vi "Select Script Mode and Run Script.vi"(7 "script name":string, 8 "error in (no error)":errorcluster, 11 "Semiconductor Module Context":T1) -> (0 "error out":errorcluster, 2 "HSDIO GEN Sessions Out":refnum<k15>[](array[refnum]), 3 "Semiconductor Module Context Out":T1)   [LabVIEW 2013]
uses:
  <vilib>/NI_TestStand_SemiconductorModule/NI_TestStand_Semiconductor_Module.lvlibp/PinMap/General/SemiconductorModuleContext.ctl
  <instrlib>/niHSDIO/niHSDIO.llb/niHSDIO_ctl Generation Mode Values (Ring).ctl
  <vilib>/NI_TestStand_SemiconductorModule/NI_TestStand_Semiconductor_Module.lvlibp
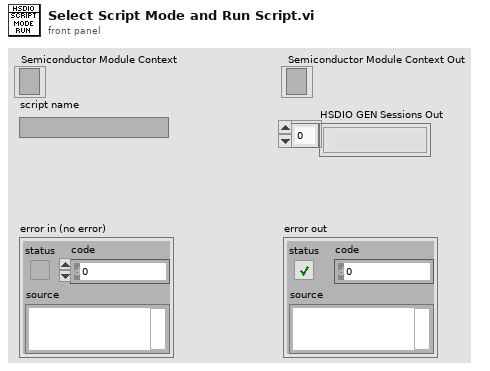
[diagram p1: front panel]
types:
  T1 = typedef "NI_TestStand_Semiconductor_Module.lvlibp/SemiconductorModuleContext.ctl" = refnum<k7>
  T2 = typedef "niHSDIO_ctl Generation Mode Values (Ring).ctl" = i32
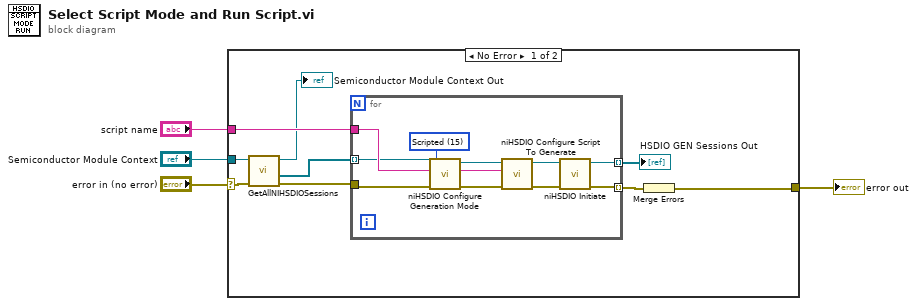
[diagram p0: block diagram]
diagram:
  n1 = case shown="No Error" "error in (no error)" {
    selector: "error in (no error)" -> [w8 w24]
    tunnel: "Semiconductor Module Context" -> [w13 _]
    tunnel: "script name" -> [w11 _]
    tunnel: [w9 w24] -> w2
    frame No Error {
      n2 = call <vilib>:"GetAllNIHSDIOSessions.vi"("error in (no error)"=w8, "Semiconductor Module Context"=w13) -> ("error out"=w7:errorcluster, "Generation Sessions"=w12:refnum<k15>[], "Semiconductor Module Context Out"=→"Semiconductor Module Context Out":T1)  [unwired: 6 in, 1 out]
      n3 = for {
        tunnel: w7 -> [w17]
        tunnel: w12 -> [w16] mode=indexing
        tunnel: w11 -> [w23]
        tunnel: [w21] -> w10 mode=indexing
        tunnel: [w20] -> w5 mode=indexing
        w18 = T2 15 items=["Waveform"=14, "Scripted"=15] ("generation mode (waveform)")
        n4 = call <instrlib>:"niHSDIO Configure Generation Mode.vi"("error in (no error)"=w17, "generation mode (waveform)"=w18, "instrument handle"=w16) -> ("error out"=w15:errorcluster, "instrument handle out"=w14:refnum<k15>)  [unwired: 7 in]
        n5 = call <instrlib>:"niHSDIO Configure Script To Generate.vi"("error in (no error)"=w15, "script name"=w23, "instrument handle"=w14) -> ("error out"=w19:errorcluster, "instrument handle out"=w22:refnum<k15>)  [unwired: 7 in]
        n6 = call <instrlib>:"niHSDIO Initiate.vi"("error in (no error)"=w19, "instrument handle"=w22) -> ("error out"=w21:errorcluster, "instrument handle out"=w20:refnum<k15>)  [unwired: 8 in]
      }
      "HSDIO GEN Sessions Out" <- w5
      n7 = Merge Errors(w10) -> (w9:errorcluster)
    }
    frame Error {
    }
  }
  "error out" <- w2
